vi "GetAcqusition.vi"(8 "error in (no error)":errorcluster, 10 "ModuleID":i32, 11 "ScopePluginsBase in":refnum<class "ScopePluginsBase.lvclass">) -> (0 "error out":errorcluster, 3 "ScopePluginsBase out":refnum<class "ScopePluginsBase.lvclass">)   [LabVIEW 2018, in "ScopePlugins.lvlib" / "ScopePluginsBase.lvclass"]
uses:
  ScopePluginsBase.lvclass
  ScopePluginsBase.lvclass/ScopePluginsBase.ctl
  Accessors/Read Acquisition.vi
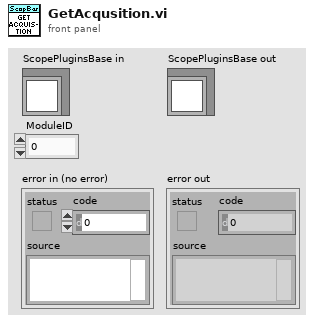
[diagram p1: front panel]
types:
  T1 = typedef "ScopePlugins.lvlib/Acquisition.ctl" = cluster{"StartTime":dbl, "Type":enum16{"Normal", "PeakDetect", "HighRes", "Envelope", "Average"}, "NumPointsMin":i32, "RecordLength":i32, "SampleRate":dbl, "TimePerRecord":dbl, "SamplingMode ":enum16{"Real Time", "Equivalent Time", "Segment", "Real Time Peak Detect", "Real Time High Resolution", "Peak Detect Segment", "High Resolution Segment"}, "Interpolation":enum16{"No Interpolation", "sin(x)/x", "linear", "1 Point sin(x)/x", "2 Point sin(x)/x", "4 Point sin(x)/x", "8 Point sin(x)/x", "16 Point sin(x)/x"}, "NumAverages":i32, "Resolution":enum16{"Auto", "Bits 9", "Bits 10", "Bits 11", "Bits 12"}, "EnableAveraging":bool, "Continuous":bool}
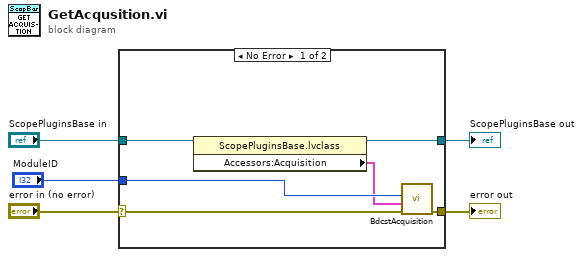
[diagram p0: block diagram]
diagram:
  n1 = case shown="No Error" "error in (no error)" {
    selector: "error in (no error)" -> [w7 w13]
    tunnel: [w6 w13] -> w4
    tunnel: [w10 w12] -> w2
    tunnel: "ScopePluginsBase in" -> [w11 w12]
    tunnel: "ModuleID" -> [w9 _]
    frame No Error {
      n2 = property class="ScopePluginsBase.lvclass"(reference=w11) -> (reference out=w10:refnum<class "ScopePluginsBase.lvclass">, "Accessors:Acquisition"=w8:T1)  [unwired: 1 in, 1 out]
      n3 = call "BdcstAcquisition.vi"("error in (no error)"=w7, "Acquisition"=w8, "ModuleID"=w9) -> ("error out"=w6:errorcluster)  [unwired: 8 in]
    }
    frame Error {
    }
  }
  "error out" <- w4
  "ScopePluginsBase out" <- w2
